vi "Configure Measurement Path_HSDIO_PFI.vi"(5 "Test_Configuration":enum16{"Relay_Off", "Relay_On"}(ring), 10 "Pins":string[](array[string])=["SW1", "SW2"], 11 "Semiconductor Module Context":T1) -> (0 "error out":errorcluster)   [LabVIEW 2013]
uses:
  <vilib>/NI_TestStand_SemiconductorModule/NI_TestStand_Semiconductor_Module.lvlibp/PinMap/General/SemiconductorModuleContext.ctl
  <vilib>/NI_TestStand_SemiconductorModule/NI_TestStand_Semiconductor_Module.lvlibp/PinMap/HSDIO/PinsToNIHSDIOSessions.vi
  <vilib>/NI_TestStand_SemiconductorModule/NI_TestStand_Semiconductor_Module.lvlibp
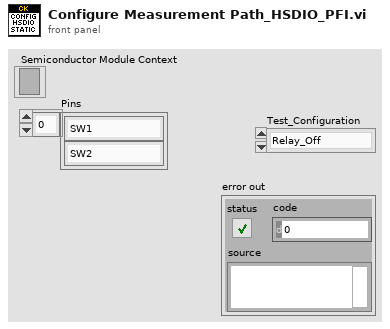
[diagram p1: front panel]
types:
  T1 = typedef "NI_TestStand_Semiconductor_Module.lvlibp/SemiconductorModuleContext.ctl" = refnum<k7>
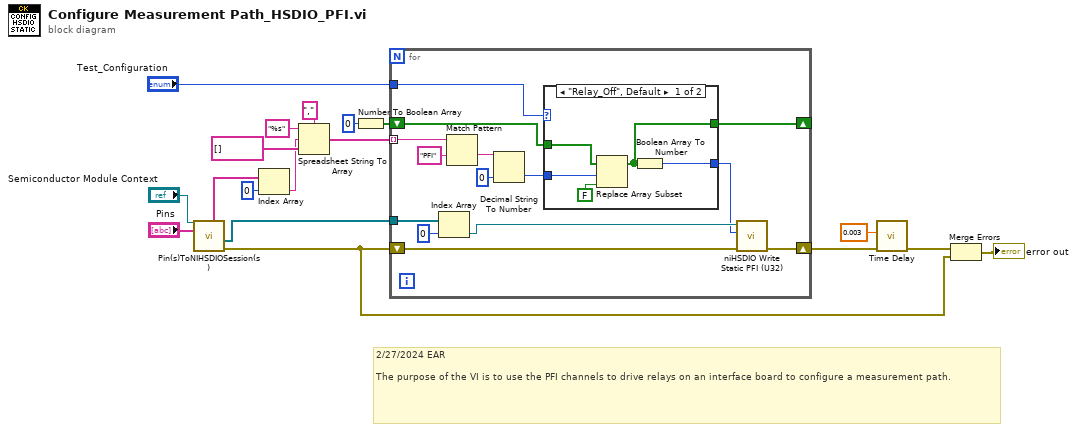
[diagram p0: block diagram]
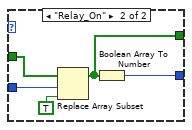
[diagram p2: hidden frame]
diagram:
  # "2/27/2024 EAR\n\nThe purpose of the VI is to use the PFI channels to drive relays on an interface board to configure a measurement path."
  n1 = call-poly <vilib>:"Pin(s)ToNIHSDIOSession(s).vi"("Pins"="Pins", "Semiconductor Module Context"="Semiconductor Module Context") -> ("error out"=w13:errorcluster, "Generation Sessions"=w18:refnum<k15>[], "Channel Lists"=w9:string[])  [unwired: 4 in, 3 out]
  n2 = Index Array(array=w9, index=0) -> (element=w7:string)
  n3 = Spreadsheet String To Array(delimiter (Tab)=",", format string="%s", spreadsheet string=w7, array type (2D Dbl)=string[] []) -> (array=w6:string[])
  n4 = Number To Boolean Array(number=0 ("Numeric")) -> (Boolean array=w4:bool[])
  n5 = for {
    tunnel: w6 -> [w27] mode=indexing
    tunnel: w18 -> [w25]
    tunnel: "Test_Configuration" -> [w28]
    shift-right: [w20] -> _
    shift-left: w4 -> [w19]
    shift-right: [w22] -> w2
    shift-left: w13 -> [w26]
    n6 = Index Array(array=w25, index=0) -> (element=w24:refnum<k15>)
    n7 = Match Pattern(string=w27, regular expression="PFI") -> (after substring=w31:string)  [unwired: 1 in, 3 out]
    n8 = Decimal String To Number(string=w31, default (0L)=0 ("default (0 I32)")) -> (number=w32:i32)  [unwired: 1 in, 1 out]
    n9 = case shown="\"Relay_Off\", Default" w28 {
      tunnel: w32 -> [w36 w40]
      tunnel: [w34 w41] -> w21
      tunnel: w19 -> [w35 w39]
      tunnel: [w33 w38] -> w20
      frame "Relay_Off", Default {
        n10 = Replace Array Subset(array=w35, new element=FALSE ("Boolean"), index=w36) -> (w33:bool[])
        n11 = Boolean Array To Number(Boolean array=w33) -> (number=w34:u32)
      }
      frame "Relay_On" {
        n12 = Replace Array Subset(array=w39, new element=TRUE ("Boolean"), index=w40) -> (w38:bool[])
        n13 = Boolean Array To Number(Boolean array=w38) -> (number=w41:u32)
      }
    }
    n14 = call <instrlib>:"niHSDIO Write Static PFI (U32).vi"("error in (no error)"=w26, "write data (0x0000)"=w21, "instrument handle"=w24) -> ("error out"=w22:errorcluster)  [unwired: 7 in, 1 out]
  }
  n15 = call "Time Delay"("error in (no error)"=w2, "Delay Time (s)"=0.003) -> ("error out"=w1:errorcluster)  [unwired: 9 in]
  n16 = Merge Errors(w1, w13) -> (→"error out":errorcluster)
